vi "GlobalCount.vi"() -> ()   [LabVIEW 2010]
panel:
  out "count":dbl
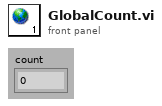
[diagram p1: front panel]
diagram:
